vi "New LSM9DS1 IMU.vi"(8 "error in (no error)":errorcluster, 11 "I2C in":refnum<class "LINX I2C.lvclass">) -> (0 "error out":errorcluster, 3 "LSM9DS1 IMU out":refnum<class "LSM9DS1 IMU.lvclass">)   [LabVIEW 2020, in "LSM9DS1 IMU.lvclass"]
uses:
  LSM9DS1 IMU.lvclass
  LINX I2C/LINX I2C.lvclass
  LSM9DS1 IMU.lvclass/LSM9DS1 IMU.ctl
  Write Accel & Gyro I2C.vi
  Write Magnetometer I2C.vi
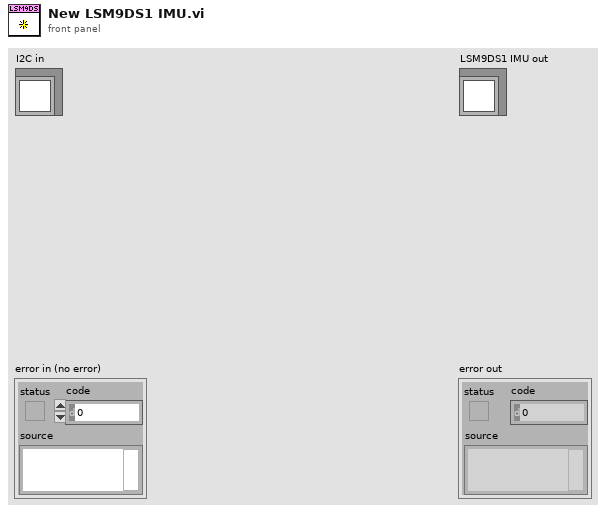
[diagram p1: front panel]
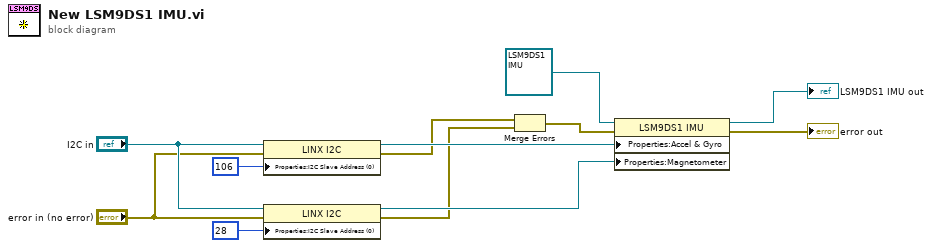
[diagram p0: block diagram]
diagram:
  n1 = property class="LINX I2C"(reference="I2C in", error in="error in (no error)", "Properties:I2C Slave Address (0)"=u8 106 ("I2C Slave Address (0)")) -> (reference out=w8:refnum<class "LINX I2C.lvclass">, error out=w5:errorcluster)
  n2 = property class="LINX I2C"(reference="I2C in", error in="error in (no error)", "Properties:I2C Slave Address (0)"=u8 28 ("I2C Slave Address (0)")) -> (reference out=w7:refnum<class "LINX I2C.lvclass">, error out=w6:errorcluster)
  n3 = Merge Errors(w5, w6) -> (w4:errorcluster)
  n4 = property class="LSM9DS1 IMU"(reference=refnum<class "LSM9DS1 IMU.lvclass"> refnum ("LSM9DS1 IMU out 2"), error in=w4, "Properties:Accel & Gyro"=w8, "Properties:Magnetometer"=w7) -> (reference out=→"LSM9DS1 IMU out":refnum<class "LSM9DS1 IMU.lvclass">, error out=→"error out":errorcluster)
